vi "Control1.vi"() -> ()   [LabVIEW 2018]
panel:
  in  "QUIT":bool
  in  "File Close Action":enum16{"Prompt", "Keep", "Archive", "Trash"}(ring)
  in  "File Information":T1={"Project"=enum."H2TC", "SubFolder"="Temp Dependence", "Filename (Meas. Description)"="200C", "Measurement number"=0}
  in  "Wait time (ms)":i32=250
  in  "Vi Selection":bool[](array[boolean])=[TRUE, TRUE, TRUE, TRUE, FALSE]
  in  "stop":bool
  # "spectrometer"
  # "powermeter"
  # "Sensors"
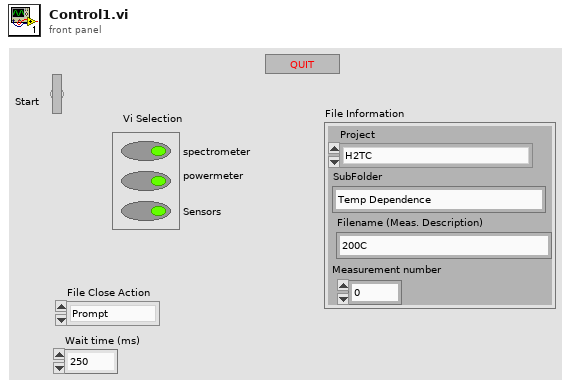
[diagram p1: front panel]
types:
  T1 = cluster{"Project":enum16{"H2TC", "VAPOR1"}, "SubFolder":string, "Filename (Meas. Description)":string, "Measurement number":i32}
  T2 = enum32{"Invalid", "Standard", "Closed", "Hidden", "Minimized", "Maximized"}
  T3 = cluster{"VI out":refnum<vi>, "error out":errorcluster, "Output cluster refnum":refnum<vi>, enum16{"TestVi", "TestVi_2", "TestVi_3"}}
  T4 = enum32{"Bad", "Idle", "Run top level", "Running"}
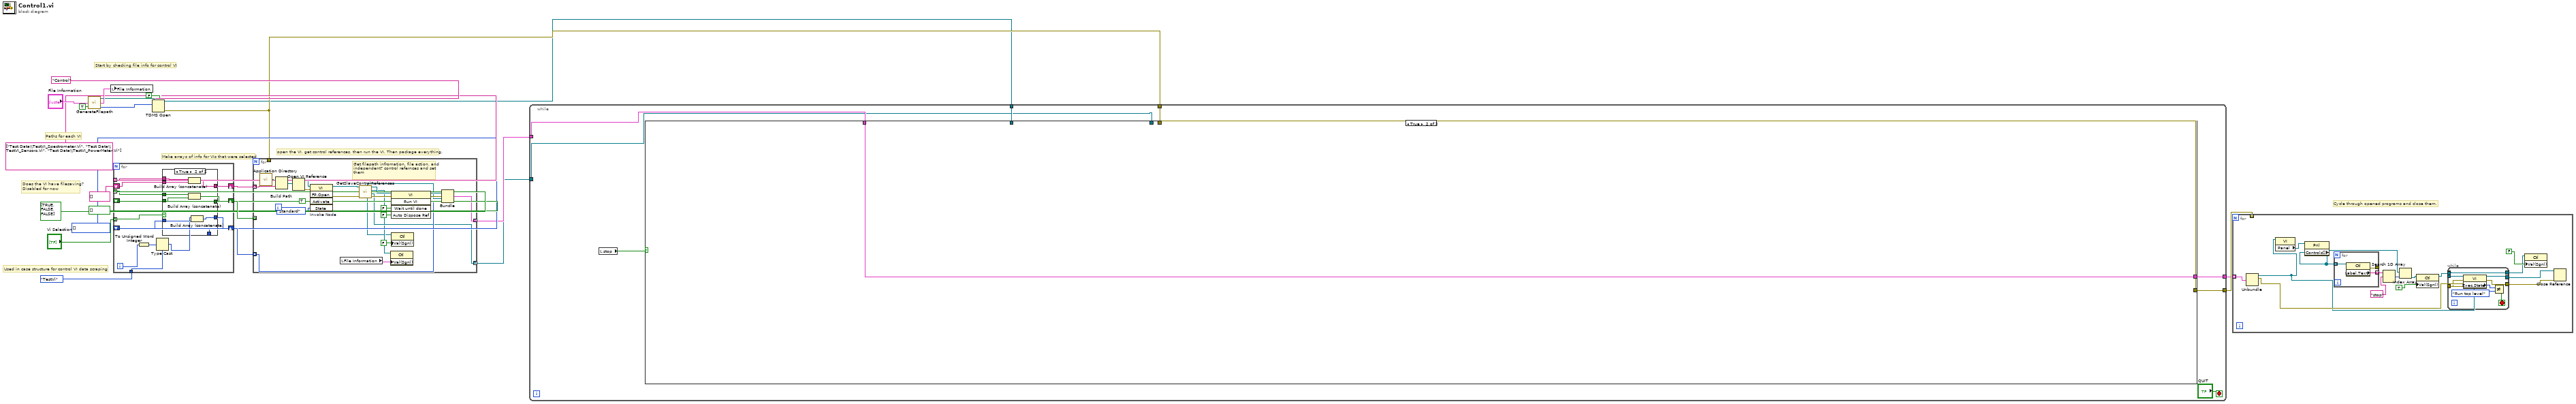
[diagram p0: block diagram]
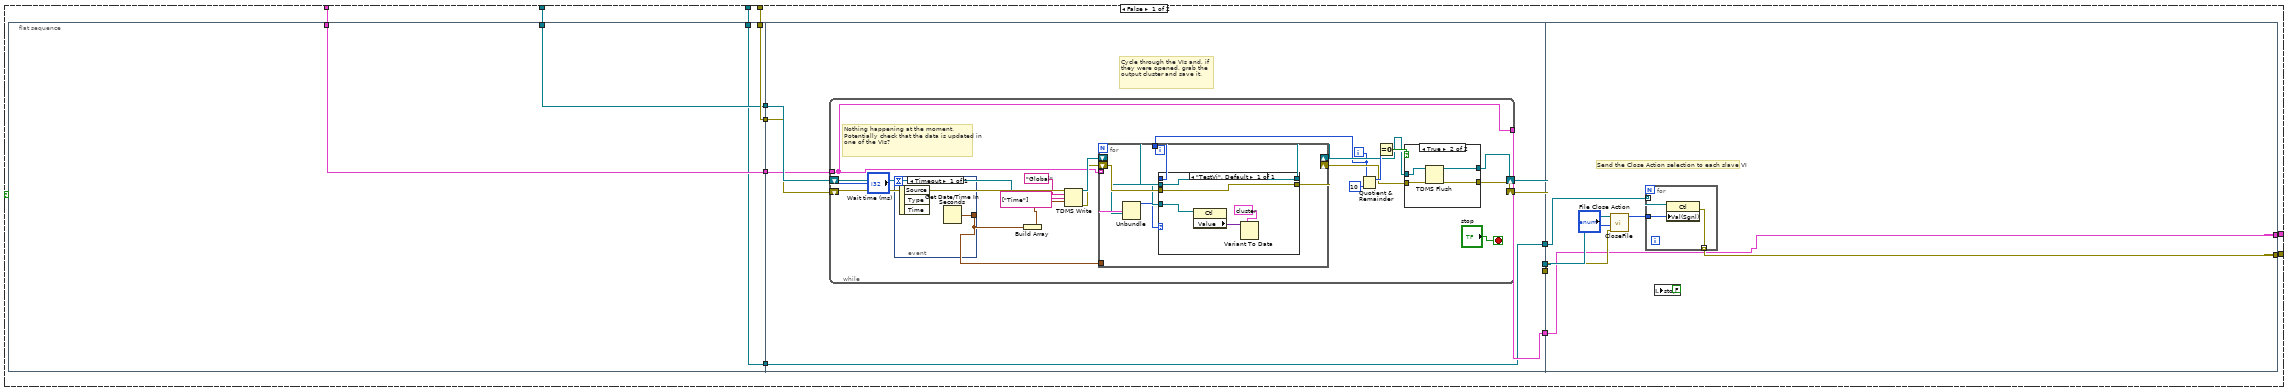
[diagram p3: hidden frame]
diagram:
  w5 = enum16{"TestVi", "TestVi_2", "TestVi_3"}[] [] items=["TestVi", "TestVi_2", "TestVi_3"]
  # "Start by checking file info for control VI"
  # "open the VI, get control references, then run the VI. Then package everything."
  # "Make arrays of info for VIs that were selected"
  # "Paths for each VI"
  # "Does the VI have filesaving?\nDisabled for now"
  # "Used in case structure for control VI data scraping"
  # "Cycle through opened programs and close them."
  n1 = call "GenerateFilepath.vi"("Check for file?"=TRUE, "File Information"="File Information", "Instrument"="Control") -> ("File Action"=w19:i32, "File Information Out"=w21:T1, "File Path Out"=w18:path)
  n2 = local write "File Information"(w21) -> ()
  n3 = for {
    tunnel: bool[] [TRUE, FALSE, FALSE] ("Vi Selection 2") -> [w32] mode=indexing
    tunnel: "Vi Selection" -> [w33] mode=indexing
    tunnel: string[] ["Test Data\\TestVI_Spectrometer.Vi", "Test Data\\TestVI_Sensors.Vi", "Test Data\\TestVI_PowerMeter.Vi"] ("name or relative path") -> [w29] mode=indexing
    tunnel: enum16{"TestVi", "TestVi_2", "TestVi_3"}."TestVi" -> [w35]
    shift-right: [w31] -> w15
    shift-left: bool[] [] -> [w30]
    shift-right: [w28] -> w16
    shift-left: string[] [] -> [w27]
    shift-right: [w25] -> w14
    shift-left: w5 -> [w24]
    i -> [w34]
    n4 = To Unsigned Word Integer(number=w34) -> (unsigned 16bit integer=w36:u16)
    n5 = Type Cast(type=w35, x=w36) -> (*(type *) &x=w26:enum16{"TestVi", "TestVi_2", "TestVi_3"})
    n6 = case shown="True" w33 {
      tunnel: w32 -> [_ w48]
      tunnel: [w39 w47] -> w31
      tunnel: w30 -> [w39 w46]
      tunnel: w29 -> [_ w45]
      tunnel: [w38 w44] -> w28
      tunnel: w27 -> [w38 w43]
      tunnel: w26 -> [_ w41]
      tunnel: [w37 w40] -> w25
      tunnel: w24 -> [w37 w42]
      frame False {
      }
      frame True {
        n7 = Build Array (concatenate)(w45, w43) -> (w44:string[])
        n8 = Build Array (concatenate)(w48, w46) -> (w47:bool[])
        n9 = Build Array (concatenate)(w41, w42) -> (w40:enum16{"TestVi", "TestVi_2", "TestVi_3"}[])
      }
    }
  }
  n10 = TDMS Open(5:FALSE ("create index file? (T)"), 10:w19, 11:w18) -> (0:w4:errorcluster, 3:w3:refnum<k34>)  [unwired: 4 in]
  n11 = for {
    tunnel: w16 -> [w71] mode=indexing
    tunnel: w15 -> [_] mode=indexing
    tunnel: [w64] -> w2 mode=indexing
    tunnel: w14 -> [w57] mode=indexing
    tunnel: [w56] -> w1 mode=indexing
    tunnel: w4 -> [_]
    # "Get filepath infromation, file action, and independent? control refernces and set them"
    n12 = call <vilib>:"Application Directory.vi"() -> ("Application Directory"=w69:path)
    n13 = Build Path(base path=w69, name or relative path=w71) -> (appended path=w67:path)
    n14 = Open VI Reference(vi path=w67) -> (vi reference=w70:refnum<vi>, error out=w68:errorcluster)  [unwired: 5 in]
    n15 = invoke on="Invoke Node" class="VI" method="FP.Open"(reference=w70, error in=w68, "Activate"=TRUE ("Activate?"), "State"=T2."Standard") -> (reference out=w59:refnum<vi>, error out=w58:errorcluster)  [unwired: 1 in, 3 out]
    n16 = local read "File Information"() -> (w53:T1)
    n17 = call "GetSlaveControlReferences.vi"("error in (no error)"=w58, "VI in"=w59) -> ("error out"=w62:errorcluster, "File Close Action Refnum"=w56:refnum<vi>, "File info Refnum"=w54:refnum<vi>, "VI out"=w63:refnum<vi>, "Indepedent? Control"=w52:refnum<vi>, "Output cluster refnum"=w55:refnum<vi>)  [unwired: 4 in]
    n18 = property class="Ctl"(reference=w54, "Val(Sgnl)"=w53) -> ()  [unwired: 1 in, 2 out]
    n19 = invoke class="VI" method="Run VI"(reference=w63, error in=w62, "Wait until done"=FALSE ("Wait Until Done"), "Auto Dispose Ref"=FALSE ("Auto Dispose Reference")) -> (reference out=w66:refnum<vi>, error out=w65:errorcluster)  [unwired: 1 in, 3 out]
    n20 = property class="Ctl"(reference=w52, "Val(Sgnl)"=FALSE) -> ()  [unwired: 1 in, 2 out]
    n21 = Bundle("VI out"=w66, "error out"=w65, "Output cluster refnum"=w55, w57) -> (w64:T3)  [unwired: 1 in]
  }
  n22 = while {
    tunnel: [w77] -> w23
    tunnel: [w76] -> w22
    tunnel: w4 -> [w75]
    tunnel: w3 -> [w74]
    tunnel: w2 -> [w73]
    tunnel: w1 -> [w72]
    stop <- "QUIT" stop-if-true
    n23 = local read "stop"() -> (w79:bool)
    n24 = case shown="True" w79 {
      tunnel: [w85 w155] -> w77
      tunnel: [w84 w156] -> w76
      tunnel: w75 -> [w83 w155]
      tunnel: w74 -> [w82 _]
      tunnel: w73 -> [w81 w156]
      tunnel: w72 -> [w80 _]
      frame False {
        n25 = flat-sequence {
          tunnel: [w96] -> w93
          tunnel: [w97] -> w92
          tunnel: [w95] -> w91
          tunnel: [w94] -> w90
          tunnel: w83 -> [w97]
          tunnel: w82 -> [w96]
          tunnel: w81 -> [w95]
          tunnel: w80 -> [w94]
          tunnel: [w103] -> w89
          tunnel: [w104] -> w88
          tunnel: [w99] -> w87
          tunnel: w93 -> [w102]
          tunnel: w92 -> [w101]
          tunnel: w91 -> [w100]
          tunnel: [w98] -> w86
          tunnel: w90 -> [w98]
          tunnel: w89 -> [w147]
          tunnel: w88 -> [w148]
          tunnel: w87 -> [w144]
          tunnel: w86 -> [w149]
          tunnel: [w145] -> w85
          tunnel: [w144] -> w84
          frame #0 {
          }
          frame #1 {
            # "Cycle through the VIs and, if they were opened, grab the output cluster and save it."
            n26 = while {
              shift-right: [w111] -> w104
              shift-left: w102 -> [w117]
              shift-right: [w110] -> w103
              shift-left: w101 -> [w118]
              tunnel: w100 -> [w105]
              tunnel: [w105] -> w99
              i -> [w106]
              stop <- "stop" stop-if-true
              # "Nothing happening at the moment. Potentially check that the data is updated in one of the VIs?"
              n27 = event shown="[0] Timeout" {
                selector: _ -> [_]
                dyn-events: _ -> [_]
                timeout: "Wait time (ms)" -> [_]
                tunnel: [w124] -> w108
                event Timeout {
                  n28 = event-data() -> ()  [unwired: 1 in, 3 out]
                  n29 = Get Date/Time In Seconds() -> (seconds since 1Jan1904=w124:timestamp)
                }
              }
              n30 = Build Array(w108) -> (w116:timestamp[])
              n31 = TDMS Write(0:w117, 5:"Global" ("group name in (Untitled)"), 7:string[] ["Time"] ("channel name(s) in (Untitled)"), 9:w116, 11:w118) -> (4:w113:refnum<k34>, 15:w112:errorcluster)  [unwired: 1 in, 2 out]
              n32 = for {
                tunnel: w105 -> [w132] mode=indexing
                shift-right: [w129] -> w120
                shift-left: w113 -> [w131]
                shift-right: [w128] -> w109
                shift-left: w112 -> [w130]
                tunnel: w108 -> [_]
                tunnel: w106 -> [w125]
                n33 = Unbundle(w132) -> ("Output cluster refnum"=w127:refnum<vi>, w126:enum16{"TestVi", "TestVi_2", "TestVi_3"})  [unwired: 2 out]
                n34 = case shown="\"TestVi\", Default" w126 {
                  tunnel: w127 -> [w136]
                  tunnel: w131 -> [w135]
                  tunnel: w130 -> [w134]
                  tunnel: [w135] -> w129
                  tunnel: [w134] -> w128
                  tunnel: w125 -> [_]
                  frame "TestVi", Default {
                    n35 = property class="Ctl"(reference=w136) -> ("Value"=w137:variant)  [unwired: 1 in, 2 out]
                    n36 = Variant To Data(type=cluster{"Sine with Uniform Noise":dynamicdata} {"Sine with Uniform Noise"=[{"t0"=timestamp(3610577859.0026608 s since 1904-01-01), "dt"=0.001, "Y"=[-0.16133839886461693], "attributes"=variant("NI_ChannelName"=variant(string "Sine with Uniform Noise"), "NI_ExpIsRelativeTime"=variant(bool FALSE), "NI_ExpStartTimeStamp"=variant(timestamp timestamp(3610577841.968661 s since 1904-01-01)), "NI_ExpTimeStamp"=variant(timestamp timestamp(3610577859.0026608 s since 1904-01-01)), "NI_ExpXDimension"=variant(string "t"))}]} ("output cluster"), Variant=w137) -> ()  [unwired: 1 in, 2 out]
                  }
                }
              }
              n37 = Quotient & Remainder(x=w106, y=10) -> (x-y*floor(x/y)=w121:i32)  [unwired: 1 out]
              n38 = Equal To 0?(x=w121) -> (x = 0?=w122:bool)
              n39 = case shown="True" w122 {
                tunnel: [w138 w143] -> w111
                tunnel: [w139 w142] -> w110
                tunnel: w109 -> [w139 w141]
                tunnel: w120 -> [w138 w140]
                frame False {
                }
                frame True {
                  n40 = TDMS Flush(4:w141, 7:w140) -> (0:w142:errorcluster, 3:w143:refnum<k34>)
                }
              }
            }
          }
          frame #2 {
            # "Send the Close Action selection to each slave VI"
            n41 = call "CloseFile.vi"("error in (no error)"=w147, "Action"="File Close Action", "Refnum in"=w148) -> ("File Close action out"=w146:enum16{"Prompt", "Keep", "Archive", "Trash"})  [unwired: 8 in]
            n42 = for {
              tunnel: w149 -> [w154] mode=indexing
              tunnel: [w153] -> w145 mode=indexing
              tunnel: w146 -> [w152]
              n43 = property class="Ctl"(reference=w154, "Val(Sgnl)"=w152) -> (error out=w153:errorcluster)  [unwired: 1 in, 1 out]
            }
            n44 = local write "stop"(FALSE ("stop")) -> ()
          }
        }
      }
      frame True {
      }
    }
  }
  n45 = for {
    tunnel: w22 -> [w170] mode=indexing
    tunnel: w23 -> [_] mode=indexing
    n46 = Unbundle(w170) -> ("VI out"=w158:refnum<vi>, "error out"=w169:errorcluster)  [unwired: 2 out]
    n47 = property class="VI"(reference=w158) -> ("Panel"=w159:refnum<vi>)  [unwired: 1 in, 2 out]
    n48 = property class="Pnl"(reference=w159) -> ("Controls[]"=w157:refnum<vi>[])  [unwired: 1 in, 2 out]
    n49 = for {
      tunnel: w157 -> [w174] mode=indexing
      tunnel: [w173] -> w166 mode=indexing
      tunnel: [w172] -> _
      n50 = property class="Ctl"(reference=w174) -> (error out=w172:errorcluster, "Label.Text"=w173:string)  [unwired: 1 in, 1 out]
    }
    n51 = Search 1D Array(1D array=w166, element="stop") -> (index of element=w165:i32)  [unwired: 1 in]
    n52 = Index Array(array=w157, index=w165) -> (element=w167:refnum<vi>)
    n53 = property class="Ctl"(reference=w167, "Val(Sgnl)"=TRUE) -> (reference out=w162:refnum<vi>)  [unwired: 1 in, 1 out]
    n54 = while {
      tunnel: w158 -> [w182]
      tunnel: [w181] -> w171
      tunnel: w169 -> [w177]
      tunnel: [w176] -> w168
      tunnel: [w175] -> _
      tunnel: w162 -> [w175]
      tunnel: [w175] -> w160
      stop <- w180 stop-if-true
      n55 = property class="VI"(reference=w182, error in=w177) -> (reference out=w181:refnum<vi>, error out=w176:errorcluster, "Exec.State"=w179:T4)
      n56 = Not Equal?(x=w179, y=T4."Run top level" ("Execution:State 2")) -> (x != y?=w180:bool)
    }
    n57 = property class="Ctl"(reference=w160, "Val(Sgnl)"=FALSE) -> ()  [unwired: 1 in, 2 out]
    n58 = Close Reference(reference=w171, error in (no error)=w168) -> ()  [unwired: 1 out]
  }
